vi "CalibrateSLM.vi"(11 "Experiment Root":path) -> ()   [LabVIEW 2019]
uses:
  <vilib>/Analysis/1siggen.llb/Ramp Pattern by Samples.vi
  <vilib>/Utility/file.llb/Write Delimited Spreadsheet (DBL).vi
  <vilib>/Analysis/1siggen.llb/Ramp Pattern by Delta.vi
  <vilib>/Utility/file.llb/Write Delimited Spreadsheet (I64).vi
  <vilib>/Utility/file.llb/Read Delimited Spreadsheet (DBL).vi
  <vilib>/Analysis/NI_AALPro.lvlib
  <vilib>/Analysis/NI_AALBase.lvlib
panel:
  in  "Mask B Transmission":cluster{i32[], i32[]}[](array[cluster])
  in  "Mask A Transmission":cluster{i32[], i32[]}[](array[cluster])
  out "Current Voltage 2":dbl min=100.0 max=200.0
  out "Current Mask 2":string
  in  "Px to WL Array":dbl[](array[numeric])
  out "Current Mask":string
  out "Current Voltage":dbl min=100.0 max=200.0
  in  "OK":bool
  in  "Tab Control":enum32{"Wavelength", "Transmission", "Phase"}(tab)
  in  "Read Spectrum":bool
  out "Current Spectrum":cluster{"Wavelength array":dbl[], i32[]}(graph)
  in  "Open Px Array":dbl[](array[numeric])
  in  "Mask A Open Count":dbl
  in  "Maximize Array":bool
  in  "Corresponding WL Array":dbl[](array[numeric])
  out "Wavelength vs. Pixel":dbl[](graph)
  in  "Fit Px to WL":bool
  in  "Maximize All":bool
  in  "Minimize All":bool
  out "Mask B Transmission":i32[][](graph)
  out "Mask A Transmission":i32[][](graph)
  in  "Transmission A":bool
  in  "Step":dbl
  in  "Start":dbl
  in  "End":dbl=1.0
  out "Mask A":dbl
  out "Mask B":dbl
  in  "Ending Pixel":dbl
  in  "Starting Pixel":dbl
  out "Phase":cluster{"Ramp Pattern":dbl[], "phase out":dbl[]}(graph)
  out "Current Pixel":dbl
  in  "Phase 2":bool
  out "Transmission":cluster{dbl[], dbl[]}[](graph)
  # "Counts"
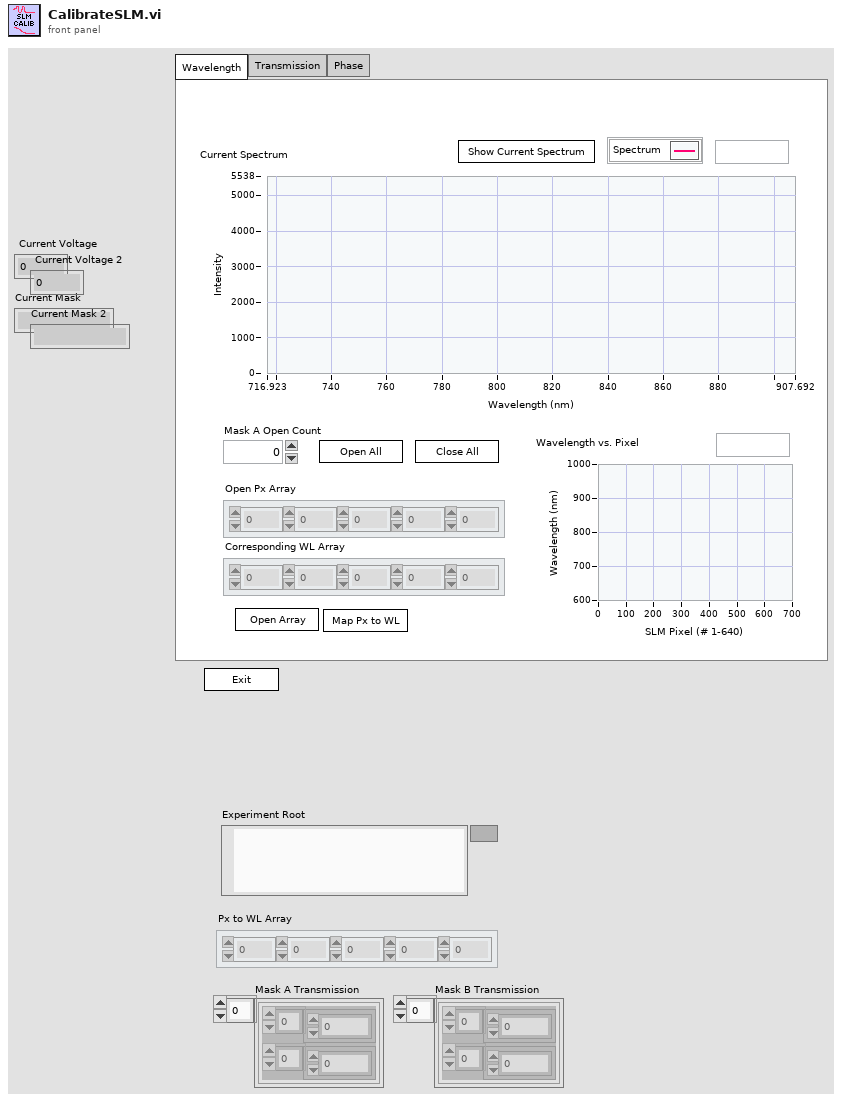
[diagram p1: front panel]
types:
  T1 = enum32{"Invalid", "Standard", "Closed", "Hidden", "Minimized", "Maximized"}
  T2 = enum32{"invalid app kind", "Development System", "Run Time System", "Student Edition", "Embedded LabVIEW", "Evaluation", "Custom"}
  T3 = cluster{"Core":cluster{"Current VI Reference":refnum<vi>, "Close Panel on Exit?":bool}, "Your Boolean data":bool, "SLM GUID":string, "Px to WL Array":dbl[], "Mask A Transmission":cluster{i32[], i32[]}[], "Mask B Transmission":cluster{i32[], i32[]}[], "Experiment Root":path}
  T4 = cluster{"Current VI Reference":refnum<vi>, "Close Panel on Exit?":bool}
  T5 = cluster{"type":enum16{"minimum", "maximum"}, "x":i32, "y":dbl}[]
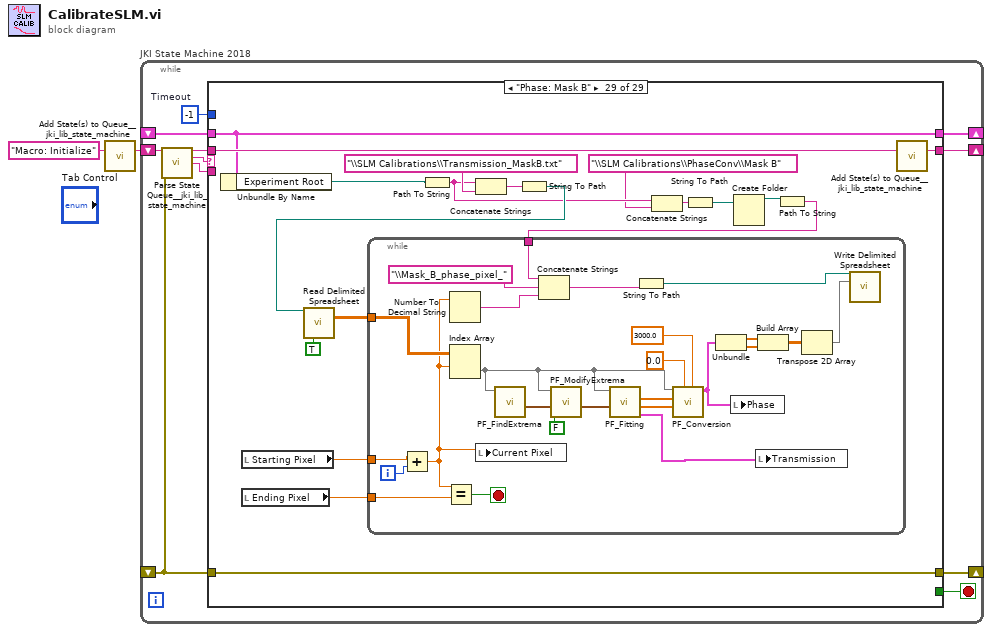
[diagram p0: block diagram]
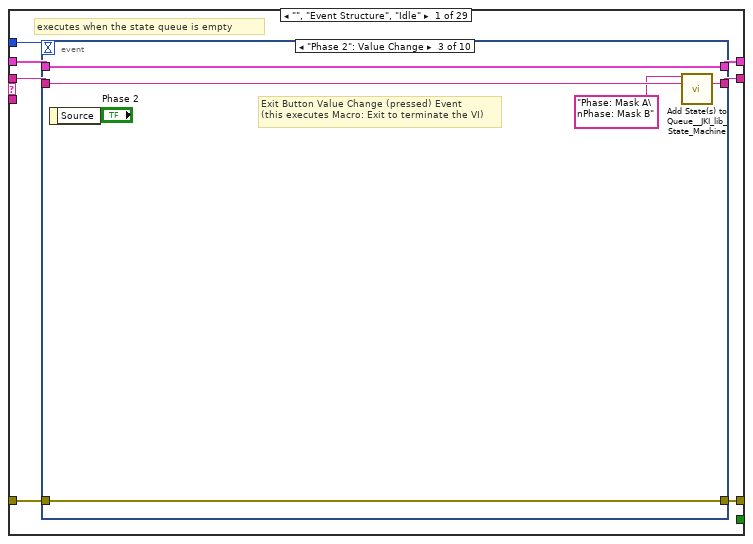
[diagram p2: hidden frame]
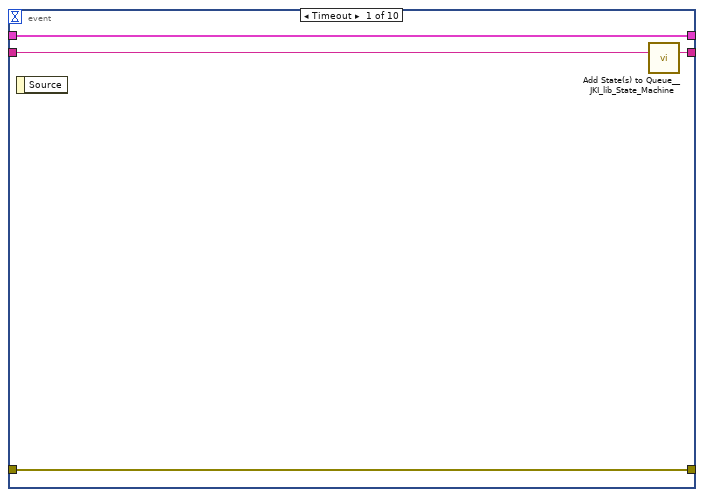
[diagram p3: hidden frame]
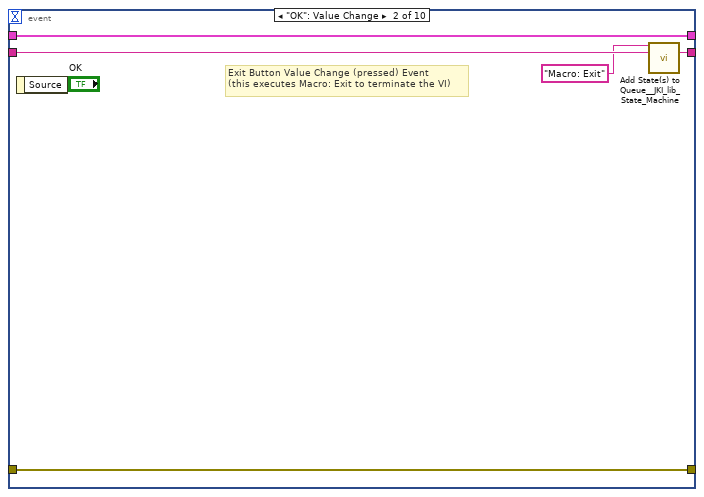
[diagram p4: hidden frame]
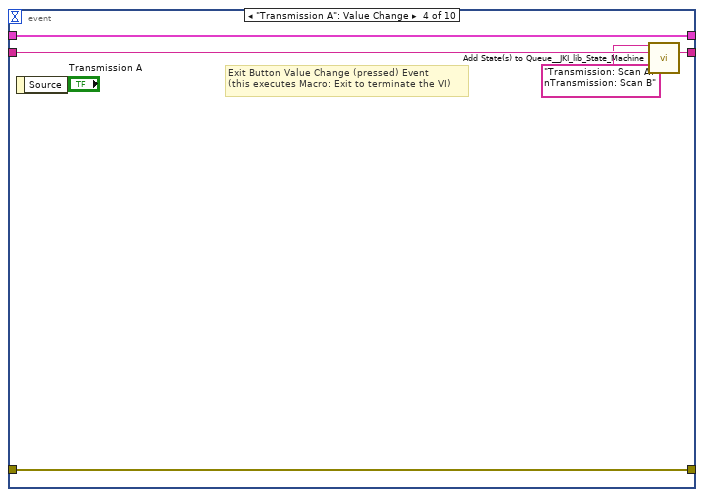
[diagram p5: hidden frame]
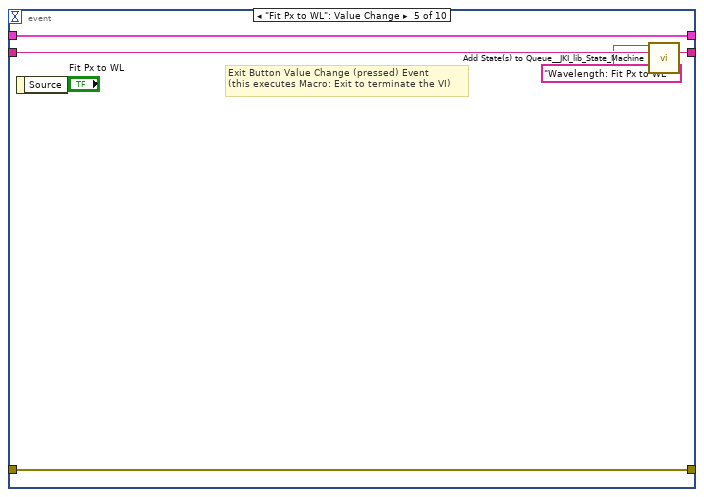
[diagram p6: hidden frame]
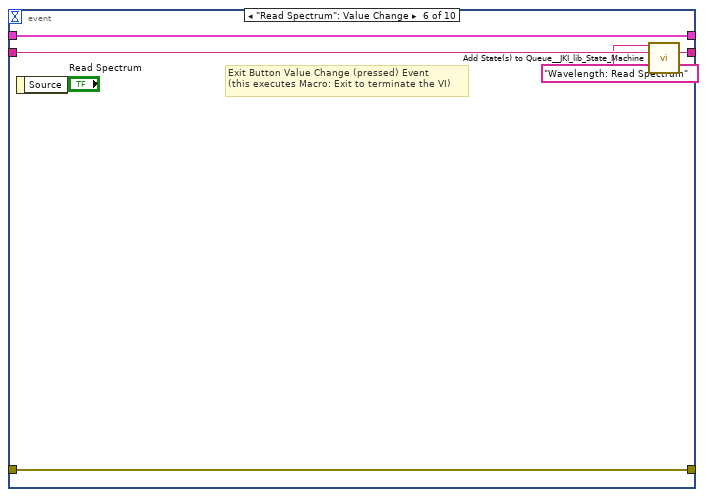
[diagram p7: hidden frame]
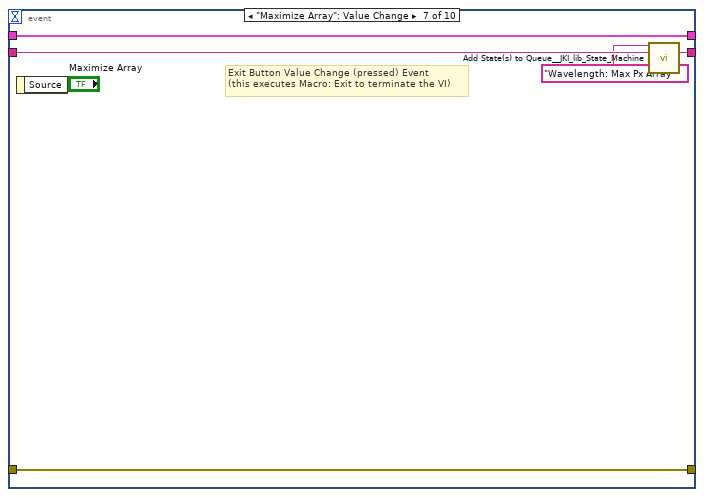
[diagram p8: hidden frame]
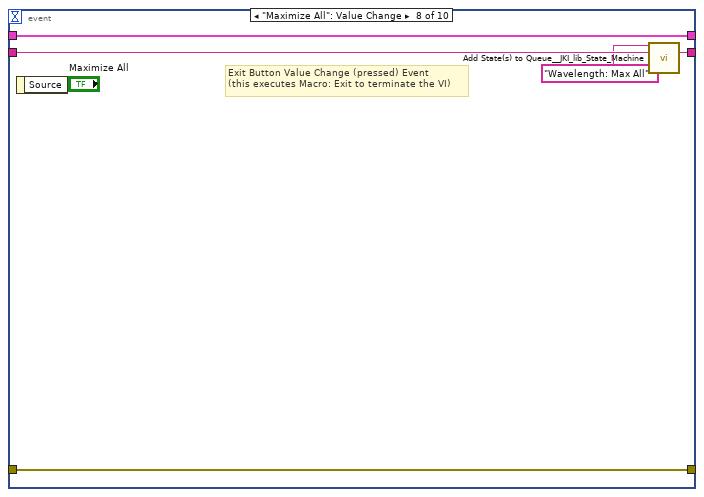
[diagram p9: hidden frame]
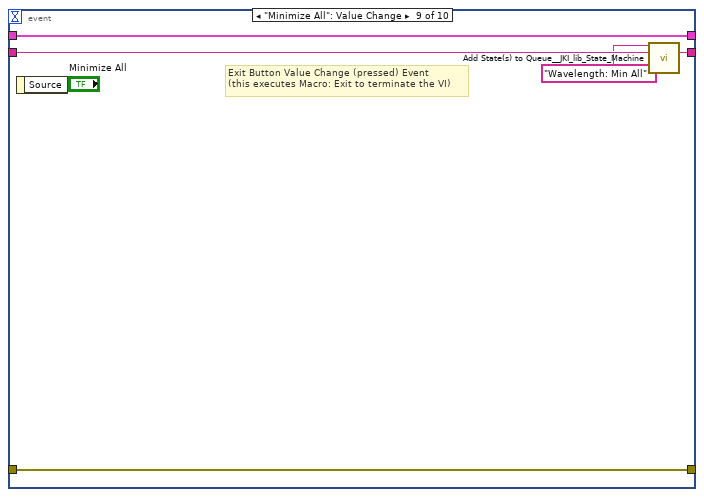
[diagram p10: hidden frame]
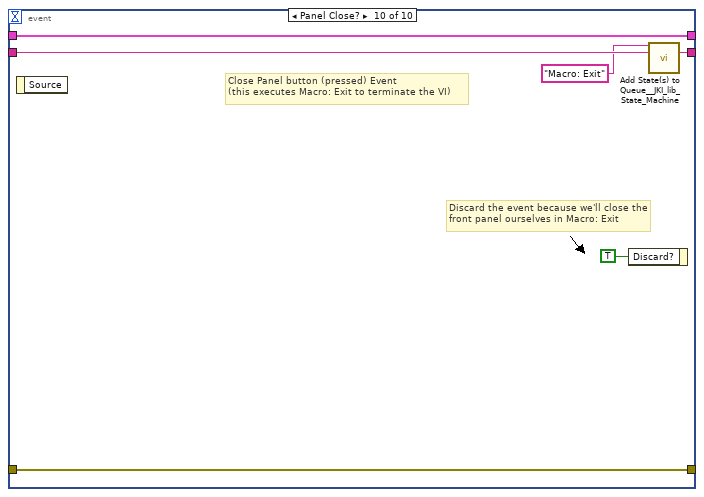
[diagram p11: hidden frame]
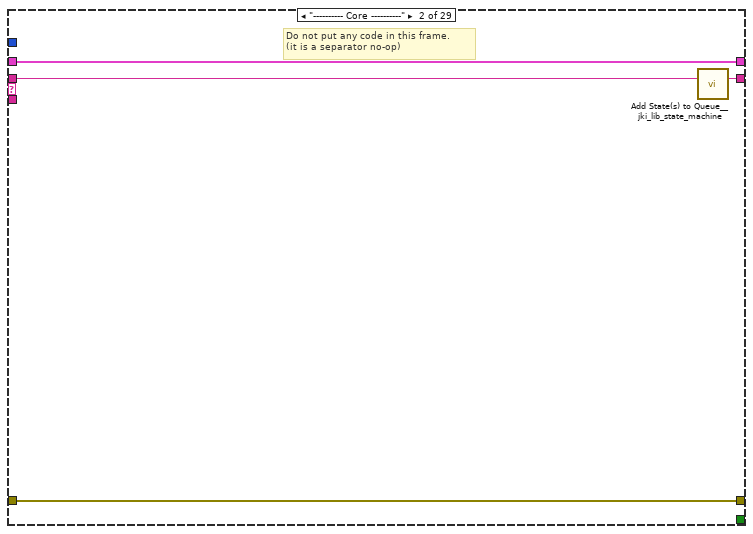
[diagram p12: hidden frame]
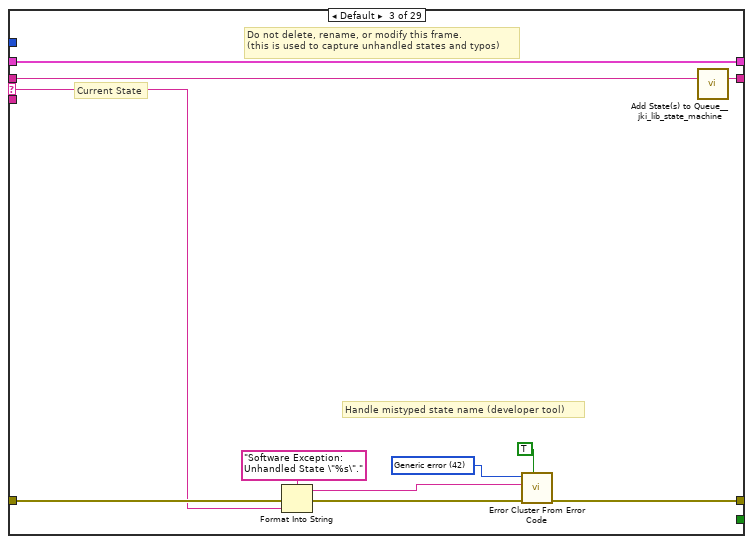
[diagram p13: hidden frame]
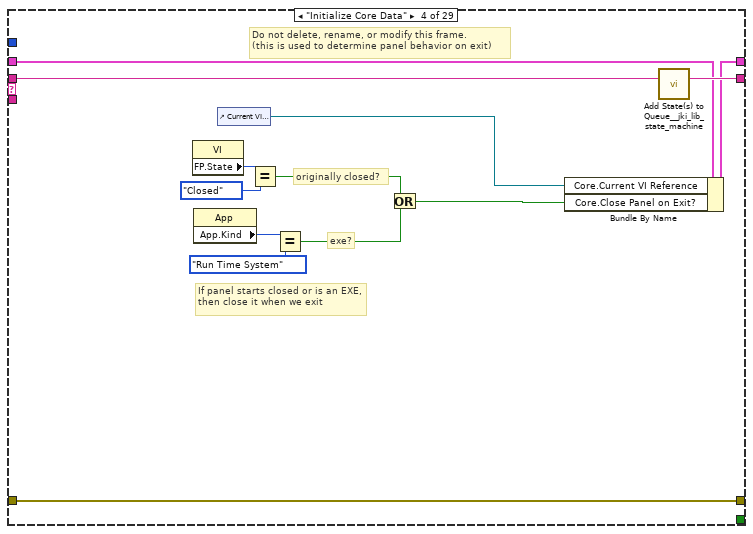
[diagram p14: hidden frame]
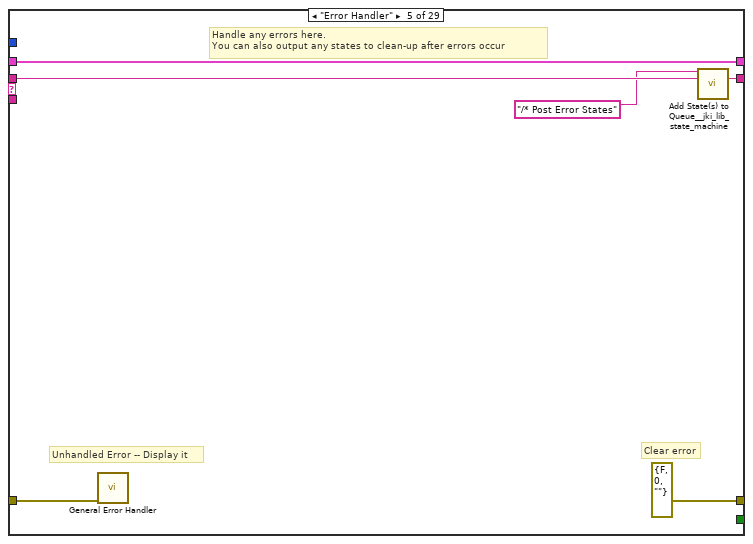
[diagram p15: hidden frame]
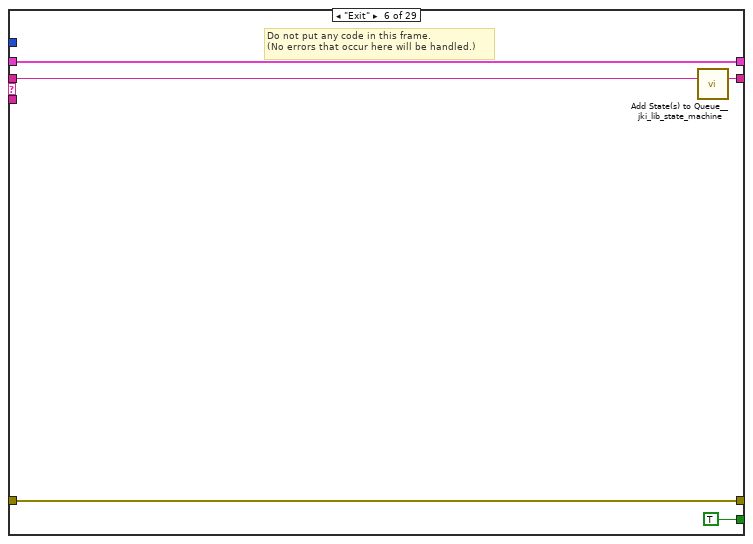
[diagram p16: hidden frame]
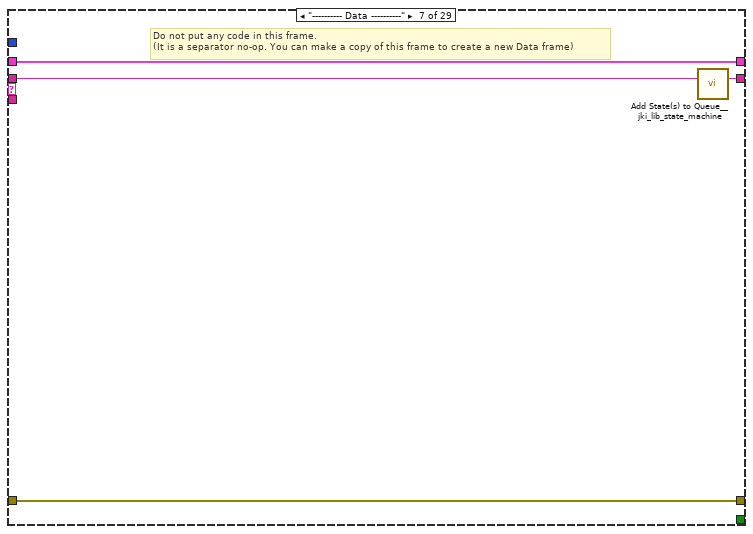
[diagram p17: hidden frame]
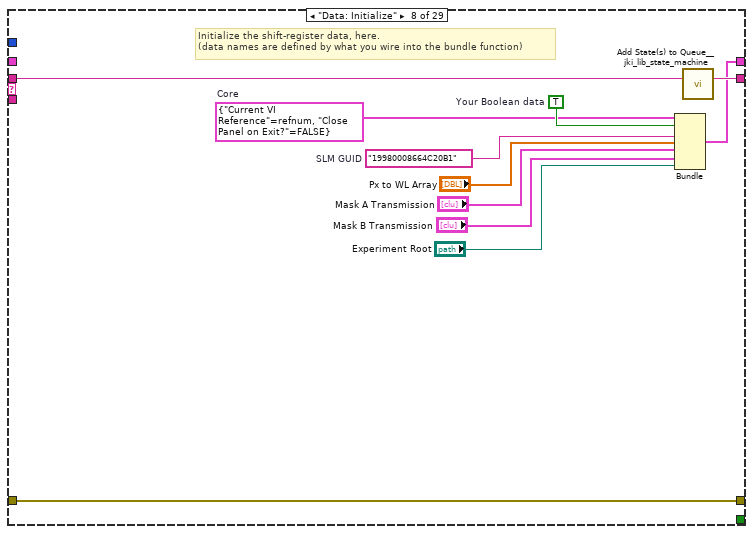
[diagram p18: hidden frame]
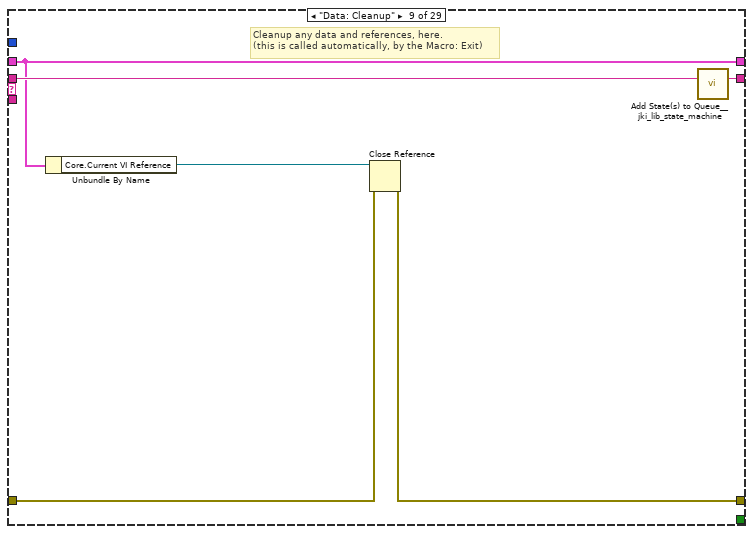
[diagram p19: hidden frame]
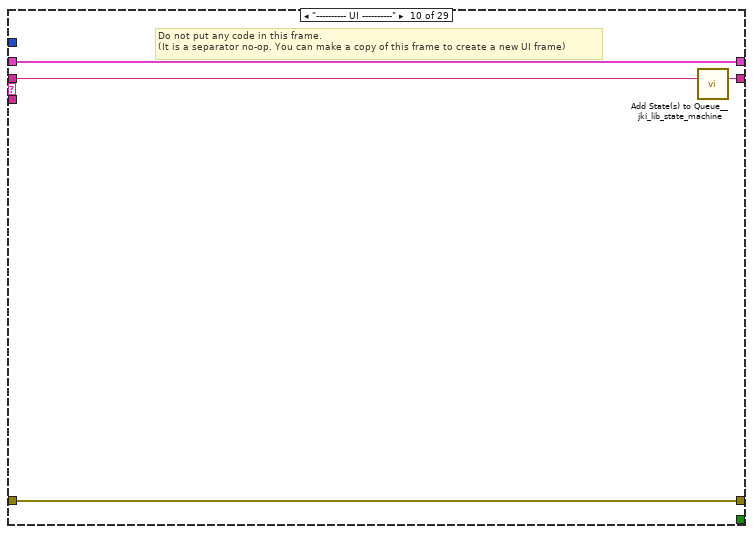
[diagram p20: hidden frame]
diagram:
  n1 = call <vilib>:"Add State(s) to Queue__jki_lib_state_machine.vi"("State(s) in (\"\")"="Macro: Initialize") -> ("States Out"=w2:string)  [unwired: 14 in]
  n2 = while "JKI State Machine 2018" {
    shift-right: [w6] -> _
    shift-left: _ -> [w5]
    shift-right: [w9] -> _
    shift-left: _ -> [w3]
    shift-right: [w8] -> _
    shift-left: w2 -> [w10]
    stop <- w7 stop-if-true
    w4 = -1  # Timeout
    n3 = call <vilib>:"Parse State Queue__jki_lib_state_machine.vi"("State Queue"=w10, "Error In (no error)"=w3) -> ("Remaining States"=w12:string, "Current State"=w13:string, "Arguments"=w11:string)  [unwired: 11 in]
    n4 = case shown="\"Phase: Mask B\"" w13 {
      selector: w13 -> [_ _ w75 _ _ _ _ _ _ _ _ _ _ _ _ _ _ _ _ _ _ _ _ _ _ _ _ _ _]
      tunnel: w12 -> [w20 w74 w79 w98 w104 w109 w113 w124 w130 w134 w138 w144 w155 w224 w229 w239 w243 w248 w262 w288 w296 w312 w324 w341 w386 w418 w422 w440 w483]
      tunnel: w11 -> [_ _ _ _ _ _ _ _ _ _ _ w139 w149 _ _ _ _ _ _ _ _ _ _ _ _ _ _ _ _]
      tunnel: w5 -> [w18 w71 w77 w91 w101 w107 w110 _ w125 w131 w136 w142 w151 w221 w226 w236 w240 w245 w260 w272 w293 w309 w321 w338 w383 w415 w419 w435 w480]
      tunnel: [w17 w72 w81 w95 errorcluster {"status"=FALSE, "code"=0, "source"=""} ("error out") w106 w111 w121 w126 w132 w135 w140 w152 w222 w227 w237 w241 w246 w249 w286 w291 w307 w322 w339 w384 w416 w420 w438 w481] -> w9
      tunnel: w3 -> [w16 w72 w80 w95 w100 w106 w111 w121 w127 w132 w135 w141 w153 w222 w227 w237 w241 w246 w257 w286 w292 w308 w322 w339 w384 w416 w420 w438 w481]
      tunnel: [w19 w73 w78 w97 w103 w108 w112 w123 w129 w133 w137 w143 w154 w223 w228 w238 w242 w247 w261 w287 w295 w311 w323 w340 w385 w417 w421 w439 w482] -> w8
      tunnel: [_ _ _ _ _ TRUE _ _ _ _ _ _ _ _ _ _ _ _ _ _ _ _ _ _ _ _ _ _ _] -> w7
      tunnel: [w15 w71 w77 w96 w101 w107 w110 w122 w125 w131 w136 w142 w151 w221 w226 w236 w240 w245 w260 w274 w293 w309 w321 w338 w383 w415 w419 w435 w480] -> w6
      tunnel: w4 -> [w14 _ _ _ _ _ _ _ _ _ _ _ _ _ _ _ _ _ _ _ _ _ _ _ _ _ _ _ _]
      frame "", "Event Structure", "Idle" {
        # "executes when the state queue is empty"
        n5 = event shown="[2] \"Phase 2\": Value Change" {
          selector: _ -> [_ _ _ _ _ _ _ _ _ _]
          dyn-events: _ -> [_ _ _ _ _ _ _ _ _ _]
          timeout: w14 -> [_ _ _ _ _ _ _ _ _ _]
          tunnel: w20 -> [w24 w29 w34 w39 w44 w49 w54 w59 w64 w70]
          tunnel: [w23 w28 w33 w38 w43 w48 w53 w58 w63 w69] -> w19
          tunnel: w18 -> [w21 w26 w31 w36 w41 w46 w51 w56 w61 w67]
          tunnel: [w22 w27 w32 w37 w42 w47 w52 w57 w62 w68] -> w17
          tunnel: w16 -> [w22 w27 w32 w37 w42 w47 w52 w57 w62 w68]
          tunnel: [w21 w26 w31 w36 w41 w46 w51 w56 w61 w67] -> w15
          event Timeout {
            n6 = event-data() -> ()  [unwired: 1 in, 1 out]
            n7 = call <vilib>:"Add State(s) to Queue__JKI_lib_State_Machine.vi"("State(s) in (\"\")"=w24) -> ("States Out"=w23:string)  [unwired: 14 in]
          }
          event "OK": Value Change {
            # "Exit Button Value Change (pressed) Event\n(this executes Macro: Exit to terminate the VI)"
            n8 = event-data() -> ()  [unwired: 1 in, 1 out]
            n9 = call <vilib>:"Add State(s) to Queue__JKI_lib_State_Machine.vi"("State(s) in Front (\"\")"="Macro: Exit", "State(s) in (\"\")"=w29) -> ("States Out"=w28:string)  [unwired: 13 in]
          }
          event "Phase 2": Value Change {
            # "Exit Button Value Change (pressed) Event\n(this executes Macro: Exit to terminate the VI)"
            n10 = event-data() -> ()  [unwired: 1 in, 1 out]
            n11 = call <vilib>:"Add State(s) to Queue__JKI_lib_State_Machine.vi"("State(s) in Front (\"\")"="Phase: Mask A\nPhase: Mask B", "State(s) in (\"\")"=w34) -> ("States Out"=w33:string)  [unwired: 13 in]
          }
          event "Transmission A": Value Change {
            # "Exit Button Value Change (pressed) Event\n(this executes Macro: Exit to terminate the VI)"
            n12 = event-data() -> ()  [unwired: 1 in, 1 out]
            n13 = call <vilib>:"Add State(s) to Queue__JKI_lib_State_Machine.vi"("State(s) in Front (\"\")"="Transmission: Scan A\nTransmission: Scan B", "State(s) in (\"\")"=w39) -> ("States Out"=w38:string)  [unwired: 13 in]
          }
          event "Fit Px to WL": Value Change {
            # "Exit Button Value Change (pressed) Event\n(this executes Macro: Exit to terminate the VI)"
            n14 = event-data() -> ()  [unwired: 1 in, 1 out]
            n15 = call <vilib>:"Add State(s) to Queue__JKI_lib_State_Machine.vi"("State(s) in Front (\"\")"="Wavelength: Fit Px to WL", "State(s) in (\"\")"=w44) -> ("States Out"=w43:string)  [unwired: 13 in]
          }
          event "Read Spectrum": Value Change {
            # "Exit Button Value Change (pressed) Event\n(this executes Macro: Exit to terminate the VI)"
            n16 = event-data() -> ()  [unwired: 1 in, 1 out]
            n17 = call <vilib>:"Add State(s) to Queue__JKI_lib_State_Machine.vi"("State(s) in Front (\"\")"="Wavelength: Read Spectrum", "State(s) in (\"\")"=w49) -> ("States Out"=w48:string)  [unwired: 13 in]
          }
          event "Maximize Array": Value Change {
            # "Exit Button Value Change (pressed) Event\n(this executes Macro: Exit to terminate the VI)"
            n18 = event-data() -> ()  [unwired: 1 in, 1 out]
            n19 = call <vilib>:"Add State(s) to Queue__JKI_lib_State_Machine.vi"("State(s) in Front (\"\")"="Wavelength: Max Px Array", "State(s) in (\"\")"=w54) -> ("States Out"=w53:string)  [unwired: 13 in]
          }
          event "Maximize All": Value Change {
            # "Exit Button Value Change (pressed) Event\n(this executes Macro: Exit to terminate the VI)"
            n20 = event-data() -> ()  [unwired: 1 in, 1 out]
            n21 = call <vilib>:"Add State(s) to Queue__JKI_lib_State_Machine.vi"("State(s) in Front (\"\")"="Wavelength: Max All", "State(s) in (\"\")"=w59) -> ("States Out"=w58:string)  [unwired: 13 in]
          }
          event "Minimize All": Value Change {
            # "Exit Button Value Change (pressed) Event\n(this executes Macro: Exit to terminate the VI)"
            n22 = event-data() -> ()  [unwired: 1 in, 1 out]
            n23 = call <vilib>:"Add State(s) to Queue__JKI_lib_State_Machine.vi"("State(s) in Front (\"\")"="Wavelength: Min All", "State(s) in (\"\")"=w64) -> ("States Out"=w63:string)  [unwired: 13 in]
          }
          event Panel Close? {
            # "Discard the event because we'll close the front panel ourselves in Macro: Exit"
            # "Close Panel button (pressed) Event\n(this executes Macro: Exit to terminate the VI)"
            n24 = event-data() -> ()  [unwired: 1 in, 1 out]
            n25 = event-data("Discard?"=TRUE) -> ()  [unwired: 1 in, 1 out]
            n26 = call <vilib>:"Add State(s) to Queue__JKI_lib_State_Machine.vi"("State(s) in Front (\"\")"="Macro: Exit", "State(s) in (\"\")"=w70) -> ("States Out"=w69:string)  [unwired: 13 in]
          }
        }
      }
      frame "---------- Core ----------" {
        # "Do not put any code in this frame.\n(it is a separator no-op)"
        n27 = call <vilib>:"Add State(s) to Queue__jki_lib_state_machine.vi"("State(s) in (\"\")"=w74) -> ("States Out"=w73:string)  [unwired: 14 in]
      }
      frame Default {
        w84 = 42 items=["No error", "Argument error", "Memory is full", "Out of zone", "End of file", "File already open", "Generic file I/O error", "File not found", "File permission error", "Disk is full", "Duplicate path", "Too many files open", "System feature not enabled", "Resource file not found", "Cannot add resource", "Resource not found", "Image not found", "Image memory error", "Pen does not exist", "Config type invalid", "Config token not found", "Config parse error", "Config memory error", "Bad external code format", "Bad external code offset", "External code not present", "Null window", "Destroy window error", "Null menu", "Print aborted", "Bad print record", "Print driver error", "Windows error during printing", "Memory error during printing", "Print dialog error", "Generic print error", "Invalid device refnum", "Device not found", "Device parameter error", "Device unit error", "Cannot open device", "Device call aborted", "Generic error", "Cancelled by user", "Object ID too low", "Object ID too high", "Object not in heap", "Unknown heap", "Unknown object (invalid DefProc)", "Unknown object (DefProc not in table)", "Message out of range", "Invalid (null) method", "Unknown message", "Manager call not supported", "Bad address", "Network operation in progress", "Network operation timed out", "Connection is busy", "Network attribute not supported", "Network error", "Address in use", "System out of memory", "Connection aborted", "Connection refused", "Not connected", "Already connected", "Connection closed", "Initialization error (interapplication manager)", "Bad occurrence", "Wait on unbound occurrence handler", "Occurrence queue overflow", "Datalog type conflict", "Unused", "Unrecognized type (interapplication manager)", "Memory corrupt", "Failed to make temporary DLL", "Old CIN version", "Drag socket not found", "Failed to load drop-object", "Failed to register OLE object", "Failed to release OLE object", "Format specifier type mismatch", "Unknown format specifier", "Too few format specifiers", "Too many format specifiers", "Scan failed", "Newer CIN version", "Error converting to variant", "Runtime menu error", "Password tampered", "Variant attribute not found", "Incompatible variant data type", "Event data is not available", "Event Store is not present", "Occurrence is not found", "Event Queue is not created", "Event info is not available", "Refnum passed is NULL", "Error retrieving Class GUID", "Error retrieving CoClass GUID", "Error retrieving TypeLib GUID.", "Bad built application magic bytes.", "Specific driver is different from the specific driver associated with the Logical Name.", "There is no session opened to the class driver.", "Max Error", "MAX - Error with config objects", "MAX - Error loading configuration", "MAX - Group not supported"]
        # "Current State"
        # "Do not delete, rename, or modify this frame.\n(this is used to capture unhandled states and typos)"
        # "Handle mistyped state name (developer tool)"
        n28 = Format Into String(format string="Software Exception: Unhandled State \"%s\"." ("message"), error in=w80, w75) -> (resulting string=w83:string, error out=w82:errorcluster)  [unwired: 1 in]
        n29 = call <vilib>:"Error Cluster From Error Code.vi"("show call chain? (False)"=TRUE, "error in (no error)"=w82, "error message (\"\")"=w83, "error code (0)"=w84) -> ("error out"=w81:errorcluster)  [unwired: 5 in]
        n30 = call <vilib>:"Add State(s) to Queue__jki_lib_state_machine.vi"("State(s) in (\"\")"=w79) -> ("States Out"=w78:string)  [unwired: 14 in]
      }
      frame "Initialize Core Data" {
        # "Do not delete, rename, or modify this frame.\n(this is used to determine panel behavior on exit)"
        # "originally closed?"
        # "exe?"
        # "If panel starts closed or is an EXE, then close it when we exit"
        n31 = property class="VI"() -> ("FP.State"=w88:T1)  [unwired: 2 in, 2 out]
        n32 = property class="App"() -> ("App.Kind"=w94:T2)  [unwired: 2 in, 2 out]
        n33 = control-ref of="Current VI Reference"() -> (w89:refnum<vi>)
        n34 = Equal?(x=w88, y=T1."Closed" ("Front Panel Window:State")) -> (x = y?=w86:bool)
        n35 = Equal?(x=w94, y=T2."Run Time System" ("Application:Kind")) -> (x = y?=w92:bool)
        n36 = Or(x=w86, y=w92) -> (x .or. y?=w90:bool)
        n37 = Bundle By Name(cluster=w91, "Core.Current VI Reference"=w89, "Core.Close Panel on Exit?"=w90) -> (w96:T3)
        n38 = call <vilib>:"Add State(s) to Queue__jki_lib_state_machine.vi"("State(s) in (\"\")"=w98) -> ("States Out"=w97:string)  [unwired: 14 in]
      }
      frame "Error Handler" {
        # "Unhandled Error -- Display it"
        # "Handle any errors here.\nYou can also output any states to clean-up after errors occur"
        # "Clear error"
        n39 = call <vilib>:"General Error Handler.vi"("error in (no error)"=w100) -> ()  [unwired: 10 in, 5 out]
        n40 = call <vilib>:"Add State(s) to Queue__jki_lib_state_machine.vi"("State(s) in Front (\"\")"="/* Post Error States", "State(s) in (\"\")"=w104) -> ("States Out"=w103:string)  [unwired: 13 in]
      }
      frame "Exit" {
        # "Do not put any code in this frame.\n(No errors that occur here will be handled.)"
        n41 = call <vilib>:"Add State(s) to Queue__jki_lib_state_machine.vi"("State(s) in (\"\")"=w109) -> ("States Out"=w108:string)  [unwired: 14 in]
      }
      frame "---------- Data ----------" {
        # "Do not put any code in this frame.\n(It is a separator no-op. You can make a copy of this frame to create a new Data frame)"
        n42 = call <vilib>:"Add State(s) to Queue__jki_lib_state_machine.vi"("State(s) in (\"\")"=w113) -> ("States Out"=w112:string)  [unwired: 14 in]
      }
      frame "Data: Initialize" {
        w118 = "19980008664C20B1"  # SLM GUID
        w119 = T4 {"Current VI Reference"=refnum, "Close Panel on Exit?"=FALSE}  # Core
        w120 = TRUE  # Your Boolean data
        # "Initialize the shift-register data, here.\n(data names are defined by what you wire into the bundle function)"
        n43 = Bundle("Core"=w119, "Your Boolean data"=w120, "SLM GUID"=w118, "Px to WL Array"="Px to WL Array", "Mask A Transmission"="Mask A Transmission", "Mask B Transmission"="Mask B Transmission", "Experiment Root"="Experiment Root") -> (w122:T3)  [unwired: 1 in]
        n44 = call <vilib>:"Add State(s) to Queue__jki_lib_state_machine.vi"("State(s) in (\"\")"=w124) -> ("States Out"=w123:string)  [unwired: 14 in]
      }
      frame "Data: Cleanup" {
        # "Cleanup any data and references, here.\n(this is called automatically, by the Macro: Exit)"
        n45 = Unbundle By Name(w125) -> ("Core.Current VI Reference"=w128:refnum<vi>)
        n46 = Close Reference(reference=w128, error in (no error)=w127) -> (error out=w126:errorcluster)
        n47 = call <vilib>:"Add State(s) to Queue__jki_lib_state_machine.vi"("State(s) in (\"\")"=w130) -> ("States Out"=w129:string)  [unwired: 14 in]
      }
      frame "---------- UI ----------" {
        # "Do not put any code in this frame.\n(It is a separator no-op. You can make a copy of this frame to create a new UI frame)"
        n48 = call <vilib>:"Add State(s) to Queue__jki_lib_state_machine.vi"("State(s) in (\"\")"=w134) -> ("States Out"=w133:string)  [unwired: 14 in]
      }
      frame "UI: Initialize" {
        # "Initialize the User Interface, here.\n(this is called automatically, by the Macro: Init)"
        n49 = call <vilib>:"Add State(s) to Queue__jki_lib_state_machine.vi"("State(s) in (\"\")"=w138) -> ("States Out"=w137:string)  [unwired: 14 in]
      }
      frame "UI: Cursor Set" {
        # "Argument"
        # "Set and Unset Cursor Busy.\n(Usage: \"UI: Cursor Set >> Busy|Idle\")"
        n50 = case shown="\"Idle\", Default" w139 {
          tunnel: w141 -> [w146 w148]
          tunnel: [w145 w147] -> w140
          frame "Idle", Default {
            n51 = call <vilib>:"Unset Busy.vi"("error in (no error)"=w146) -> ("error out"=w145:errorcluster)  [unwired: 10 in]
          }
          frame "Busy" {
            n52 = call <vilib>:"Set Busy.vi"("error in (no error)"=w148) -> ("error out"=w147:errorcluster)  [unwired: 9 in, 1 out]
          }
        }
        n53 = call <vilib>:"Add State(s) to Queue__jki_lib_state_machine.vi"("State(s) in (\"\")"=w144) -> ("States Out"=w143:string)  [unwired: 14 in]
      }
      frame "UI: Front Panel State" {
        # "Argument"
        # "Set Front Panel Open or Closed\n(Usage: \"UI: Front Panel State >> Open|Close\")"
        n54 = Unbundle By Name(w151) -> ("Core.Current VI Reference"=w150:refnum<vi>)
        n55 = case shown="\"Minimize\", \"Minimized\"" w149 {
          tunnel: w153 -> [w161 w176 w187 w200 w213]
          tunnel: [w163 w177 w189 w202 w215] -> w152
          tunnel: w150 -> [w162 w174 w188 w201 w214]
          frame "Open", "Standard", Default {
            w156 = T1."Standard" ("State")
            n56 = property class="VI"(reference=w162, error in=w161) -> (reference out=w159:refnum<vi>, error out=w160:errorcluster, "FP.State"=w158:T1)
            n57 = Not Equal?(x=w158, y=w156) -> (x != y?=w157:bool)
            n58 = case shown="True" w157 {
              tunnel: [w167 w169] -> w163
              tunnel: w160 -> [w166 w169]
              tunnel: w159 -> [w165 _]
              tunnel: w156 -> [w164 _]
              frame True {
                n59 = invoke class="VI" method="FP.Open"(reference=w165, error in=w166, "Activate"=TRUE, "State"=w164) -> (error out=w167:errorcluster)  [unwired: 1 in, 4 out]
              }
              frame False {
              }
            }
          }
          frame "Close", "Closed" {
            n60 = property class="VI"(reference=w174, error in=w176) -> (reference out=w173:refnum<vi>, error out=w175:errorcluster, "FP.State"=w171:T1)
            n61 = Not Equal?(x=w171, y=T1."Closed" ("Front Panel Window:State")) -> (x != y?=w170:bool)
            n62 = case shown="True" w170 {
              tunnel: [w178 w181] -> w177
              tunnel: w175 -> [w178 w180]
              tunnel: w173 -> [_ w179]
              frame False {
              }
              frame True {
                n63 = invoke class="VI" method="FP.Close"(reference=w179, error in=w180) -> (error out=w181:errorcluster)  [unwired: 1 in, 2 out]
              }
            }
          }
          frame "Hidden", "Hide" {
            w182 = T1."Hidden" ("State")
            n64 = property class="VI"(reference=w188, error in=w187) -> (reference out=w185:refnum<vi>, error out=w186:errorcluster, "FP.State"=w184:T1)
            n65 = Not Equal?(x=w184, y=w182) -> (x != y?=w183:bool)
            n66 = case shown="True" w183 {
              tunnel: [w193 w194] -> w189
              tunnel: w186 -> [w192 w194]
              tunnel: w185 -> [w191 _]
              tunnel: w182 -> [w190 _]
              frame True {
                n67 = invoke class="VI" method="FP.Open"(reference=w191, error in=w192, "State"=w190) -> (error out=w193:errorcluster)  [unwired: 2 in, 4 out]
              }
              frame False {
              }
            }
          }
          frame "Minimize", "Minimized" {
            w195 = T1."Minimized" ("State")
            n68 = property class="VI"(reference=w201, error in=w200) -> (reference out=w198:refnum<vi>, error out=w199:errorcluster, "FP.State"=w197:T1)
            n69 = Not Equal?(x=w197, y=w195) -> (x != y?=w196:bool)
            n70 = case shown="True" w196 {
              tunnel: [w206 w207] -> w202
              tunnel: w199 -> [w205 w207]
              tunnel: w198 -> [w204 _]
              tunnel: w195 -> [w203 _]
              frame True {
                n71 = invoke class="VI" method="FP.Open"(reference=w204, error in=w205, "State"=w203) -> (error out=w206:errorcluster)  [unwired: 2 in, 4 out]
              }
              frame False {
              }
            }
          }
          frame "Maximize", "Maximized" {
            w208 = T1."Maximized" ("State")
            n72 = property class="VI"(reference=w214, error in=w213) -> (reference out=w211:refnum<vi>, error out=w212:errorcluster, "FP.State"=w210:T1)
            n73 = Not Equal?(x=w210, y=w208) -> (x != y?=w209:bool)
            n74 = case shown="True" w209 {
              tunnel: [w219 w220] -> w215
              tunnel: w212 -> [w218 w220]
              tunnel: w211 -> [w217 _]
              tunnel: w208 -> [w216 _]
              frame True {
                n75 = invoke class="VI" method="FP.Open"(reference=w217, error in=w218, "State"=w216) -> (error out=w219:errorcluster)  [unwired: 2 in, 4 out]
              }
              frame False {
              }
            }
          }
        }
        n76 = call <vilib>:"Add State(s) to Queue__jki_lib_state_machine.vi"("State(s) in (\"\")"=w155) -> ("States Out"=w154:string)  [unwired: 14 in]
      }
      frame "---------- Macro ----------" {
        # "Do not put any code in this frame.\n(It is a separator no-op. You can make a copy of this frame to create a new Macro frame)"
        n77 = call <vilib>:"Add State(s) to Queue__jki_lib_state_machine.vi"("State(s) in (\"\")"=w224) -> ("States Out"=w223:string)  [unwired: 14 in]
      }
      frame "Macro: Initialize" {
        w225 = "Data: Initialize\nInitialize Core Data\nUI: Initialize\nUI: Front Panel State >> Open"  # Data: Initialize Initialize Core Data UI: Initialize UI: Front Panel State >> Open
        # "Initialization Macro\n(This is called once, when the VI starts)"
        n78 = call <vilib>:"Add State(s) to Queue__jki_lib_state_machine.vi"("State(s) in Front (\"\")"=w225, "State(s) in (\"\")"=w229) -> ("States Out"=w228:string)  [unwired: 13 in]
      }
      frame "Macro: Exit" {
        # "Exit Macro\n(This is called once, when the VI exits)"
        n79 = Unbundle By Name(w236) -> ("Core.Close Panel on Exit?"=w235:bool)
        n80 = Select(t="UI: Front Panel State >> Close", s=w235, f="") -> (s? t:f=w232:string)
        n81 = call <vilib>:"Add State(s) to Queue__JKI_lib_State_Machine.vi"("State(s) in (\"\")"=w232, "State(s) at Back (\"\")"="Data: Cleanup\nExit") -> ("States Out"=w230:string)  [unwired: 13 in]
        n82 = call <vilib>:"Add State(s) to Queue__jki_lib_state_machine.vi"("State(s) in Front (\"\")"=w230, "State(s) in (\"\")"=w239) -> ("States Out"=w238:string)  [unwired: 13 in]
      }
      frame "---------- Wavelength ----------" {
        n83 = call <vilib>:"Add State(s) to Queue__jki_lib_state_machine.vi"("State(s) in (\"\")"=w243) -> ("States Out"=w242:string)  [unwired: 14 in]
      }
      frame "Wavelength: Read Spectrum" {
        n84 = call "USE THIS TO GET FUND FRAME.vi"() -> ("Spectrum"=→"Current Spectrum":cluster{"Wavelength array":dbl[], i32[]})  [unwired: 10 in, 1 out]
        n85 = call <vilib>:"Add State(s) to Queue__jki_lib_state_machine.vi"("State(s) in (\"\")"=w248) -> ("States Out"=w247:string)  [unwired: 14 in]
      }
      frame "Wavelength: Max Px Array" {
        w252 = u32 4095 ("count (0..4095)")
        n86 = Unbundle By Name(w260) -> ("SLM GUID"=w250:string)
        n87 = call "SLM_Direct"("error in (no error)"=w257, "count (0..4095)"=w252, "display (A or B)"=enum16{"display A", "display B"}."display A", "port (COM or GUID)"=w250) -> ("error out"=w254:errorcluster)  [unwired: 1 in, 1 out]
        n88 = call "SLM_Direct"("error in (no error)"=w254, "count (0..4095)"=w252, "display (A or B)"=enum16{"display A", "display B"}."display B", "port (COM or GUID)"=w250) -> ("error out"=w253:errorcluster)  [unwired: 1 in, 1 out]
        n89 = for {
          tunnel: w250 -> [w269]
          tunnel: "Open Px Array" -> [w267] mode=indexing
          tunnel: "Mask A Open Count" -> [w266]
          tunnel: w253 -> [w265]
          tunnel: [w264] -> w249
          n90 = call "SLM_DirectStripe"("error in (no error)"=w265, "count (0..4095)"=w266, "stripe (s)"=w267, "display (A or B)"=enum16{"display A", "display B"}."display A", "port (COM or GUID)"=w269) -> ("error out"=w264:errorcluster)  [unwired: 1 in, 1 out]
          n91 = Wait (ms)(milliseconds to wait=u32 100) -> ()  [unwired: 1 out]
        }
        n92 = call <vilib>:"Add State(s) to Queue__jki_lib_state_machine.vi"("State(s) in Front (\"\")"="Wavelength: Read Spectrum" ("State(s) in Front (\"\")"), "State(s) in (\"\")"=w262) -> ("States Out"=w261:string)  [unwired: 13 in]
      }
      frame "Wavelength: Fit Px to WL" {
        w282 = 640.0 ("end")
        n93 = Unbundle By Name(w272) -> ("Experiment Root"=w271:path)
        n94 = local read "Open Px Array"() -> (w285:dbl[])
        n95 = Path To String(path=w271) -> (string=w277:string)
        n96 = call-poly <vilib>:"Ramp Pattern.vi"("start"=1.0, "end"=w282, "samples"=w282) -> ("Ramp Pattern"=w281:dbl[])  [unwired: 7 in, 1 out]
        n97 = call <vilib>:"Linear Fit.vi"("Y"="Corresponding WL Array", "X"=w285) -> ("slope"=w280:dbl, "intercept"=w279:dbl)  [unwired: 9 in, 3 out]
        n98 = Concatenate Strings(w277, "\\SLM Calibrations\\PxtoWL.txt" ("string")) -> (w275:string)
        n99 = String To Path(string=w275) -> (path=w270:path)
        n100 = Multiply(x=w281, y=w280) -> (x*y=w278:dbl[])
        n101 = Add(x=w278, y=w279) -> (x+y=w273:dbl[])
        "Wavelength vs. Pixel" <- w273
        n102 = call-poly <vilib>:"Write Delimited Spreadsheet.vi"("file path (dialog if empty)"=w270, "1D data"=w273) -> ()  [unwired: 12 in, 2 out]
        n103 = Bundle By Name(cluster=w272, "Px to WL Array"=w273) -> (w274:T3)
        n104 = call <vilib>:"Add State(s) to Queue__jki_lib_state_machine.vi"("State(s) in (\"\")"=w288) -> ("States Out"=w287:string)  [unwired: 14 in]
      }
      frame "Wavelength: Max All" {
        # "Template Separator\n(You can make a copy of, or modify, this frame)"
        n105 = local read "Mask A Open Count"() -> (w290:dbl)
        n106 = Unbundle By Name(w293) -> ("SLM GUID"=w294:string)
        n107 = flat-sequence {
          tunnel: w294 -> [w301]
          tunnel: w292 -> [w300]
          tunnel: [w299] -> w291
          tunnel: w290 -> [w297]
          frame #0 {
            n108 = call "SLM_Direct"("error in (no error)"=w300, "count (0..4095)"=w297, "display (A or B)"=enum16{"display A", "display B"}."display A", "port (COM or GUID)"=w301) -> ("error out"=w303:errorcluster)  [unwired: 1 in, 1 out]
            n109 = call "SLM_Direct"("error in (no error)"=w303, "count (0..4095)"=u32 4095, "display (A or B)"=enum16{"display A", "display B"}."display B", "port (COM or GUID)"=w301) -> ("error out"=w299:errorcluster)  [unwired: 1 in, 1 out]
          }
          frame #1 {
            n110 = Wait (ms)(milliseconds to wait=u32 100) -> ()  [unwired: 1 out]
          }
        }
        n111 = call <vilib>:"Add State(s) to Queue__jki_lib_state_machine.vi"("State(s) in Front (\"\")"="Wavelength: Read Spectrum" ("State(s) in Front (\"\")"), "State(s) in (\"\")"=w296) -> ("States Out"=w295:string)  [unwired: 13 in]
      }
      frame "Wavelength: Min All" {
        # "Template Separator\n(You can make a copy of, or modify, this frame)"
        n112 = Unbundle By Name(w309) -> ("SLM GUID"=w310:string)
        n113 = flat-sequence {
          tunnel: w310 -> [w316]
          tunnel: w308 -> [w315]
          tunnel: [w314] -> w307
          frame #0 {
            w313 = u32 4095 ("count (0..4095)")
            n114 = call "SLM_Direct"("error in (no error)"=w315, "count (0..4095)"=w313, "display (A or B)"=enum16{"display A", "display B"}."display A", "port (COM or GUID)"=w316) -> ("error out"=w318:errorcluster)  [unwired: 1 in, 1 out]
            n115 = call "SLM_Direct"("error in (no error)"=w318, "count (0..4095)"=w313, "display (A or B)"=enum16{"display A", "display B"}."display B", "port (COM or GUID)"=w316) -> ("error out"=w314:errorcluster)  [unwired: 1 in, 1 out]
          }
          frame #1 {
            n116 = Wait (ms)(milliseconds to wait=u32 100) -> ()  [unwired: 1 out]
          }
        }
        n117 = call <vilib>:"Add State(s) to Queue__jki_lib_state_machine.vi"("State(s) in Front (\"\")"="Wavelength: Read Spectrum" ("State(s) in Front (\"\")"), "State(s) in (\"\")"=w312) -> ("States Out"=w311:string)  [unwired: 13 in]
      }
      frame "---------- Transmission ----------" {
        n118 = call <vilib>:"Add State(s) to Queue__jki_lib_state_machine.vi"("State(s) in (\"\")"=w324) -> ("States Out"=w323:string)  [unwired: 14 in]
      }
      frame "Transmission: Scan A" {
        n119 = flat-sequence {
          tunnel: w337 -> [w342]
          tunnel: [w342] -> w336
          tunnel: w336 -> [w348]
          tunnel: w335 -> [w347]
          tunnel: w332 -> [w346]
          tunnel: [w345] -> w331
          frame #0 {
            n120 = call "SLM_Direct"("count (0..4095)"=4095.0 ("Voltage counts (0-4095)"), "display (A or B)"=enum16{"display A", "display B"}."display B", "port (COM or GUID)"=w342) -> ()  [unwired: 2 in, 2 out]
          }
          frame #1 {
            n121 = for {
              tunnel: w348 -> [w352]
              tunnel: w347 -> [w351]
              tunnel: w346 -> [w350] mode=indexing
              tunnel: [w349] -> w345 mode=indexing
              n122 = flat-sequence {
                tunnel: w352 -> [w354]
                tunnel: w350 -> [w353]
                tunnel: w351 -> [w360]
                tunnel: [w357] -> w349
                frame #0 {
                  n123 = call "SLM_Direct"("count (0..4095)"=w353, "display (A or B)"=enum16{"display A", "display B"}."display A", "port (COM or GUID)"=w354) -> ()  [unwired: 2 in, 2 out]
                  "Mask A" <- w353
                }
                frame #1 {
                  n124 = Wait (ms)(milliseconds to wait=u32 100) -> ()  [unwired: 1 out]
                }
                frame #2 {
                  n125 = call "USE THIS TO GET FUND FRAME.vi"() -> ("Spectrum"=w361:cluster{"Wavelength array":dbl[], i32[]})  [unwired: 10 in, 1 out]
                  n126 = Unbundle(w361) -> ("Wavelength array"=w363:dbl[], w362:i32[])
                  n127 = for {
                    tunnel: w363 -> [w369]
                    tunnel: w362 -> [w367]
                    tunnel: [w366] -> w357 mode=indexing
                    tunnel: w360 -> [w365] mode=indexing
                    tunnel: [w364] -> w358 mode=indexing
                    i -> [w364]
                    n128 = call "Search 1D Array for Nearest LV2012 NIVerified.vi"("desired element"=w365, "1D Array"=w369) -> ("closest index"=w368:i32)  [unwired: 8 in, 1 out]
                    n129 = Index Array(array=w367, index=w368) -> (element=w366:i32)
                  }
                  n130 = Increment(x=w358) -> (x+1=w359:i32[])
                  n131 = Bundle(w359, w357) -> ()  [unwired: 1 in, 1 out]
                }
              }
            }
          }
        }
        n132 = Unbundle By Name(w338) -> ("Experiment Root"=w326:path, "Px to WL Array"=w335:dbl[], "SLM GUID"=w337:string)
        n133 = call-poly <vilib>:"Ramp Pattern.vi"("start"="Start", "end"="End", "delta"="Step") -> ("Ramp Pattern"=w332:dbl[])  [unwired: 6 in, 2 out]
        n134 = Path To String(path=w326) -> (string=w329:string)
        n135 = property on="Mask A Transmission" class="IntGraph (strict)"("XScale.Multiplier"="Step") -> ()  [unwired: 2 in, 2 out]
        n136 = Concatenate Strings(w329, "\\SLM Calibrations\\Transmission_MaskA.txt" ("string")) -> (w327:string)
        n137 = String To Path(string=w327) -> (path=w325:path)
        n138 = call-poly <vilib>:"Write Delimited Spreadsheet.vi"("file path (dialog if empty)"=w325, "2D data"=w331) -> ()  [unwired: 12 in, 2 out]
        n139 = call <vilib>:"Add State(s) to Queue__jki_lib_state_machine.vi"("State(s) in (\"\")"=w341) -> ("States Out"=w340:string)  [unwired: 14 in]
        "Mask A Transmission" <- w331
      }
      frame "Transmission: Scan B" {
        n140 = flat-sequence {
          tunnel: w382 -> [w387]
          tunnel: [w387] -> w381
          tunnel: w381 -> [w393]
          tunnel: w380 -> [w392]
          tunnel: w379 -> [w391]
          tunnel: [w390] -> w376
          frame #0 {
            n141 = call "SLM_Direct"("count (0..4095)"=4095.0 ("Voltage counts (0-4095)"), "display (A or B)"=enum16{"display A", "display B"}."display A", "port (COM or GUID)"=w387) -> ()  [unwired: 2 in, 2 out]
          }
          frame #1 {
            n142 = for {
              tunnel: w393 -> [w397]
              tunnel: w392 -> [w396]
              tunnel: w391 -> [w395] mode=indexing
              tunnel: [w394] -> w390 mode=indexing
              n143 = flat-sequence {
                tunnel: w397 -> [w399]
                tunnel: w395 -> [w398]
                tunnel: w396 -> [w405]
                tunnel: [w402] -> w394
                frame #0 {
                  n144 = call "SLM_Direct"("count (0..4095)"=w398, "display (A or B)"=enum16{"display A", "display B"}."display B", "port (COM or GUID)"=w399) -> ()  [unwired: 2 in, 2 out]
                  "Mask B" <- w398
                }
                frame #1 {
                  n145 = Wait (ms)(milliseconds to wait=u32 100) -> ()  [unwired: 1 out]
                }
                frame #2 {
                  n146 = call "USE THIS TO GET FUND FRAME.vi"() -> ("Spectrum"=w406:cluster{"Wavelength array":dbl[], i32[]})  [unwired: 10 in, 1 out]
                  n147 = Unbundle(w406) -> ("Wavelength array"=w408:dbl[], w407:i32[])
                  n148 = for {
                    tunnel: w408 -> [w414]
                    tunnel: w407 -> [w412]
                    tunnel: [w411] -> w402 mode=indexing
                    tunnel: w405 -> [w410] mode=indexing
                    tunnel: [w409] -> w403 mode=indexing
                    i -> [w409]
                    n149 = call "Search 1D Array for Nearest LV2012 NIVerified.vi"("desired element"=w410, "1D Array"=w414) -> ("closest index"=w413:i32)  [unwired: 8 in, 1 out]
                    n150 = Index Array(array=w412, index=w413) -> (element=w411:i32)
                  }
                  n151 = Increment(x=w403) -> (x+1=w404:i32[])
                  n152 = Bundle(w404, w402) -> ()  [unwired: 1 in, 1 out]
                }
              }
            }
          }
        }
        n153 = Unbundle By Name(w383) -> ("Experiment Root"=w371:path, "Px to WL Array"=w380:dbl[], "SLM GUID"=w382:string)
        n154 = local read "Start"() -> (w378:dbl)
        n155 = local read "Step"() -> (w375:dbl)
        n156 = local read "End"() -> (w377:dbl)
        n157 = call-poly <vilib>:"Ramp Pattern.vi"("start"=w378, "end"=w377, "delta"=w375) -> ("Ramp Pattern"=w379:dbl[])  [unwired: 6 in, 2 out]
        n158 = Path To String(path=w371) -> (string=w374:string)
        n159 = property on="Mask B Transmission" class="IntGraph (strict)"("XScale.Multiplier"=w375) -> ()  [unwired: 2 in, 2 out]
        n160 = Concatenate Strings(w374, "\\SLM Calibrations\\Transmission_MaskB.txt" ("string")) -> (w372:string)
        n161 = String To Path(string=w372) -> (path=w370:path)
        n162 = call-poly <vilib>:"Write Delimited Spreadsheet.vi"("file path (dialog if empty)"=w370, "2D data"=w376) -> ()  [unwired: 12 in, 2 out]
        n163 = call <vilib>:"Add State(s) to Queue__jki_lib_state_machine.vi"("State(s) in (\"\")"=w386) -> ("States Out"=w385:string)  [unwired: 14 in]
        "Mask B Transmission" <- w376
      }
      frame "Transmission: Plot/Save" {
        n164 = call <vilib>:"Add State(s) to Queue__jki_lib_state_machine.vi"("State(s) in (\"\")"=w418) -> ("States Out"=w417:string)  [unwired: 14 in]
      }
      frame "---------- Phase ----------" {
        n165 = call <vilib>:"Add State(s) to Queue__jki_lib_state_machine.vi"("State(s) in (\"\")"=w422) -> ("States Out"=w421:string)  [unwired: 14 in]
      }
      frame "Phase: Mask A" {
        n166 = Unbundle By Name(w435) -> ("Experiment Root"=w432:path)
        n167 = Path To String(path=w432) -> (string=w424:string)
        n168 = Concatenate Strings(w424, "\\SLM Calibrations\\Transmission_MaskA.txt" ("string")) -> (w433:string)
        n169 = String To Path(string=w433) -> (path=w430:path)
        n170 = call-poly <vilib>:"Read Delimited Spreadsheet.vi"("file path (dialog if empty)"=w430, "transpose? (F)"=TRUE) -> ("all rows"=w429:dbl[][])  [unwired: 8 in, 5 out]
        n171 = Concatenate Strings(w424, "\\SLM Calibrations\\PhaseConv\\Mask A" ("string")) -> (w427:string)
        n172 = String To Path(string=w427) -> (path=w426:path)
        n173 = Create Folder(path (use dialog)=w426) -> (created path=w425:path)  [unwired: 2 in, 2 out]
        n174 = Path To String(path=w425) -> (string=w423:string)
        n175 = while {
          tunnel: "Starting Pixel" -> [w456]
          tunnel: "Ending Pixel" -> [w454]
          tunnel: w429 -> [w449]
          tunnel: w423 -> [w448]
          i -> [w455]
          stop <- w453 stop-if-true
          n176 = Add(x=w456, y=w455) -> (x+y=w450:dbl)
          "Current Pixel" <- w450
          n177 = Equal?(x=w450, y=w454) -> (x = y?=w453:bool)
          n178 = Number To Decimal String(number=w450) -> (decimal integer string=w452:string)  [unwired: 1 in]
          n179 = Index Array(array=w449, index (row)=w450) -> (element=w445:dbl[])  [unwired: 1 in]
          n180 = call "PF_FindExtrema.vi"("Intensity Array"=w445) -> ("Extrema Array"=w465:T5)  [unwired: 9 in]
          n181 = Concatenate Strings(w448, "\\Mask_A_phase_pixel_" ("string"), w452) -> (w447:string)
          n182 = call "PF_ModifyExtrema.vi"("Max Voltage Range?"=FALSE, "Extremas Array In"=w465, "Intensity Array"=w445) -> ("Extremas Array Out"=w464:T5)  [unwired: 8 in]
          n183 = call "PF_Fitting.vi"("Extrema Array"=w464, "Intensity Array"=w445) -> ("Intensity"=→"Transmission":cluster{dbl[], dbl[]}[], "yFit"=w462:dbl[], "xFit"=w463:dbl[])  [unwired: 6 in]
          n184 = String To Path(string=w447) -> (path=w446:path)
          n185 = call "PF_Conversion.vi"("Intensity"=w445, "xFit"=w463, "yFit"=w462, "start"=0.0, "end"=3000.0) -> ("Phase"=w458:cluster{"Ramp Pattern":dbl[], "phase out":dbl[]})  [unwired: 5 in]
          "Phase" <- w458
          n186 = Unbundle(w458) -> ("Ramp Pattern"=w461:dbl[], "phase out"=w460:dbl[])
          n187 = Build Array(w461, w460) -> (w459:dbl[][])
          n188 = Transpose 2D Array(2D array=w459) -> (transposed array=w457:dbl[][])
          n189 = call-poly <vilib>:"Write Delimited Spreadsheet.vi"("file path (dialog if empty)"=w446, "2D data"=w457) -> ()  [unwired: 12 in, 2 out]
        }
        n190 = call <vilib>:"Add State(s) to Queue__jki_lib_state_machine.vi"("State(s) in (\"\")"=w440) -> ("States Out"=w439:string)  [unwired: 14 in]
      }
      frame "Phase: Mask B" {
        n191 = Unbundle By Name(w480) -> ("Experiment Root"=w477:path)
        n192 = local read "Starting Pixel"() -> (w468:dbl)
        n193 = local read "Ending Pixel"() -> (w467:dbl)
        n194 = Path To String(path=w477) -> (string=w470:string)
        n195 = Concatenate Strings(w470, "\\SLM Calibrations\\Transmission_MaskB.txt" ("string")) -> (w478:string)
        n196 = String To Path(string=w478) -> (path=w475:path)
        n197 = call-poly <vilib>:"Read Delimited Spreadsheet.vi"("file path (dialog if empty)"=w475, "transpose? (F)"=TRUE) -> ("all rows"=w474:dbl[][])  [unwired: 8 in, 5 out]
        n198 = Concatenate Strings(w470, "\\SLM Calibrations\\PhaseConv\\Mask B" ("string")) -> (w473:string)
        n199 = String To Path(string=w473) -> (path=w472:path)
        n200 = Create Folder(path (use dialog)=w472) -> (created path=w471:path)  [unwired: 2 in, 2 out]
        n201 = Path To String(path=w471) -> (string=w469:string)
        n202 = while {
          tunnel: w474 -> [w496]
          tunnel: w469 -> [w495]
          tunnel: w468 -> [w488]
          tunnel: w467 -> [w487]
          i -> [w500]
          stop <- w499 stop-if-true
          n203 = Add(x=w488, y=w500) -> (x+y=w490:dbl)
          n204 = Equal?(x=w490, y=w487) -> (x = y?=w499:bool)
          n205 = Number To Decimal String(number=w490) -> (decimal integer string=w498:string)  [unwired: 1 in]
          n206 = Index Array(array=w496, index (row)=w490) -> (element=w492:dbl[])  [unwired: 1 in]
          n207 = local write "Current Pixel"(w490) -> ()
          n208 = call "PF_FindExtrema.vi"("Intensity Array"=w492) -> ("Extrema Array"=w508:T5)  [unwired: 9 in]
          n209 = Concatenate Strings(w495, "\\Mask_B_phase_pixel_" ("string"), w498) -> (w494:string)
          n210 = call "PF_ModifyExtrema.vi"("Max Voltage Range?"=FALSE, "Extremas Array In"=w508, "Intensity Array"=w492) -> ("Extremas Array Out"=w507:T5)  [unwired: 8 in]
          n211 = call "PF_Fitting.vi"("Extrema Array"=w507, "Intensity Array"=w492) -> ("Intensity"=w486:cluster{dbl[], dbl[]}[], "yFit"=w505:dbl[], "xFit"=w506:dbl[])  [unwired: 6 in]
          n212 = String To Path(string=w494) -> (path=w493:path)
          n213 = call "PF_Conversion.vi"("Intensity"=w492, "xFit"=w506, "yFit"=w505, "start"=0.0, "end"=3000.0) -> ("Phase"=w489:cluster{"Ramp Pattern":dbl[], "phase out":dbl[]})  [unwired: 5 in]
          n214 = Unbundle(w489) -> ("Ramp Pattern"=w504:dbl[], "phase out"=w503:dbl[])
          n215 = local write "Phase"(w489) -> ()
          n216 = local write "Transmission"(w486) -> ()
          n217 = Build Array(w504, w503) -> (w502:dbl[][])
          n218 = Transpose 2D Array(2D array=w502) -> (transposed array=w501:dbl[][])
          n219 = call-poly <vilib>:"Write Delimited Spreadsheet.vi"("file path (dialog if empty)"=w493, "2D data"=w501) -> ()  [unwired: 12 in, 2 out]
        }
        n220 = call <vilib>:"Add State(s) to Queue__jki_lib_state_machine.vi"("State(s) in (\"\")"=w483) -> ("States Out"=w482:string)  [unwired: 14 in]
      }
    }
  }
